vi "LatchSetSpeed.vi"() -> ()   [LabVIEW 2014, in "LatchLib.lvlib"]
uses:
  LatchLib.lvlib
  <vilib>/Rock Robotics/WPI/Solenoid/WPI_SolenoidValue.ctl
panel:
  in  "LatchContainerState":bool
  in  "LatchLatchState":bool
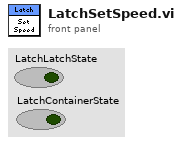
[diagram p1: front panel]
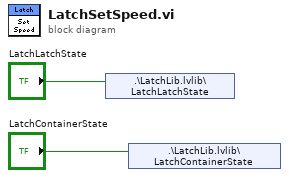
[diagram p0: block diagram]
diagram:
  n1 = shared-variable ".\\LatchLib.lvlib\\LatchLatchState"("LatchLatchState") -> ()  [unwired: 1 in, 1 out]
  n2 = shared-variable ".\\LatchLib.lvlib\\LatchContainerState"("LatchContainerState") -> ()  [unwired: 1 in, 1 out]
